vi "d_n__v1.vi"(9 "ƒÁ[n-1]":ext, 10 "z[n-1]":ext, 11 "z[n]":ext) -> (3 "d[n]":ext)   [LabVIEW 2020]
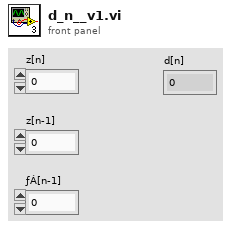
[diagram p1: front panel]
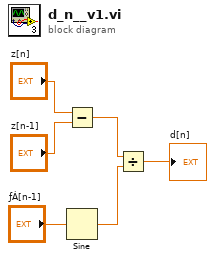
[diagram p0: block diagram]
diagram:
  n1 = Subtract(x="z[n]", y="z[n-1]") -> (x-y=w3:ext)
  n2 = Sine(x="ƒÁ[n-1]") -> (sin(x)=w2:ext)
  n3 = Divide(x=w3, y=w2) -> (x/y=→"d[n]":ext)
